vi "image_replacement.vi"(8 "buffer name":string, 10 "replacement":dbl[](array[numeric]), 11 "image in":T1(plugin-control)) -> (3 "image out":T1(plugin-control))   [LabVIEW 2017]
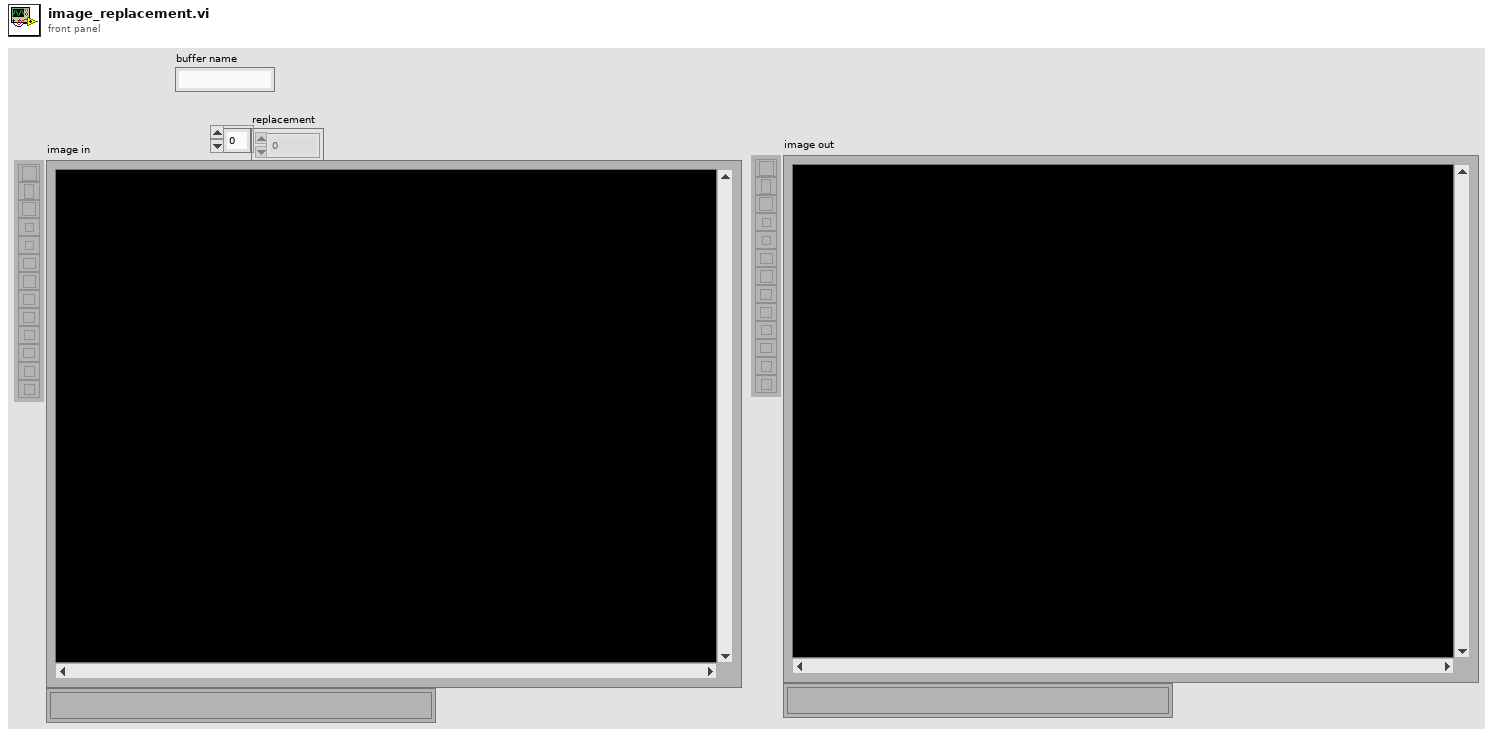
[diagram p1: front panel]
types:
  T1 = typedef "IMAQ Image.ctl" = refnum<image>
  T2 = typedef "Image Type" = u32
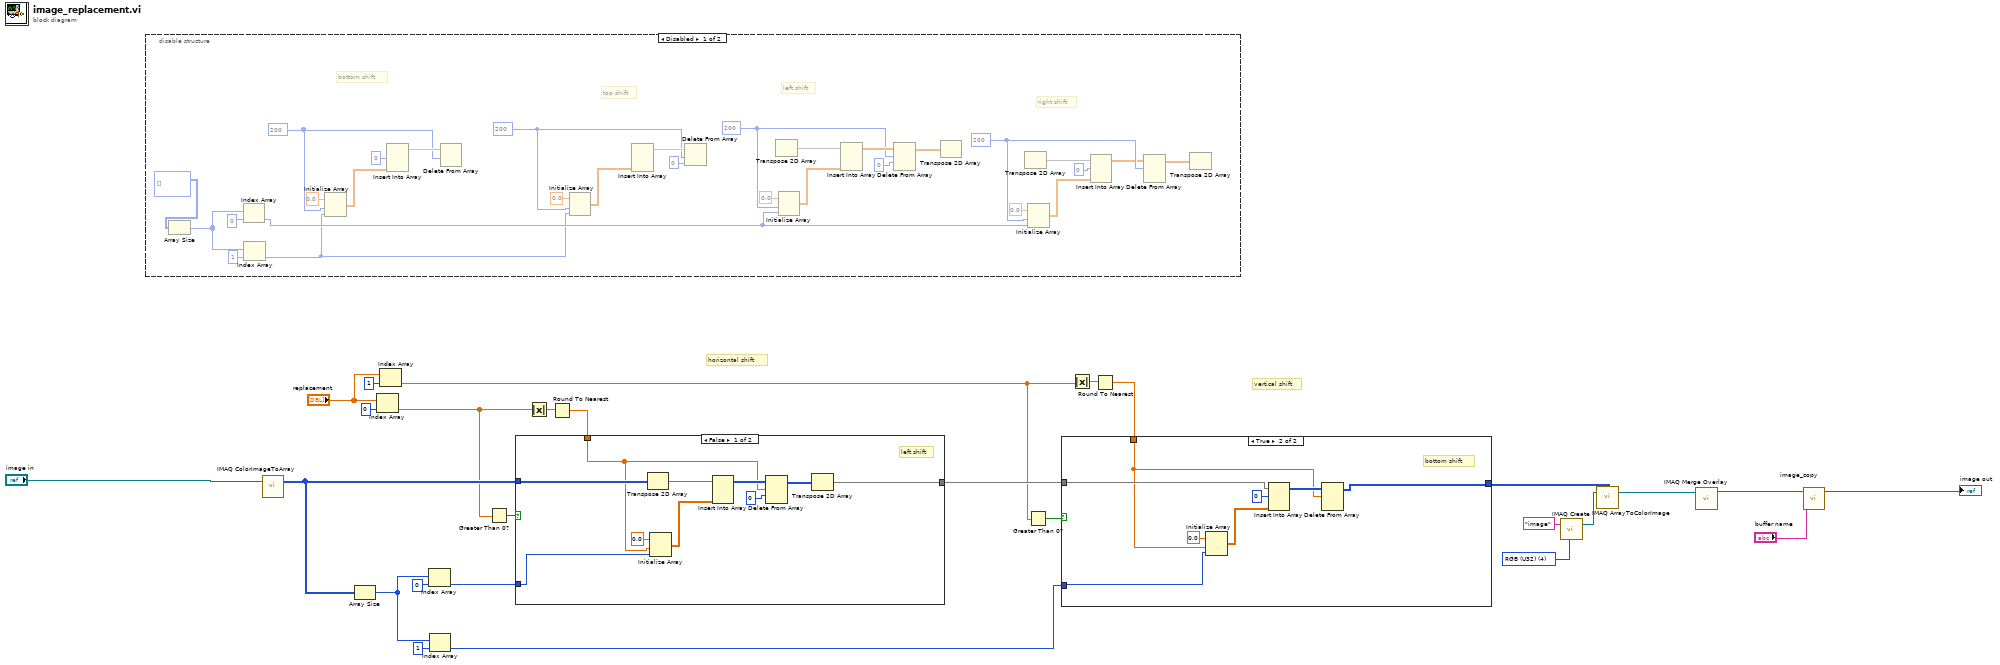
[diagram p0: block diagram]
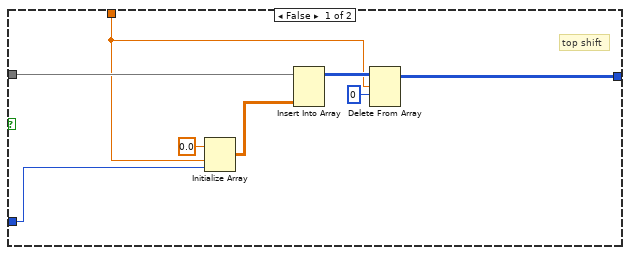
[diagram p2: hidden frame]
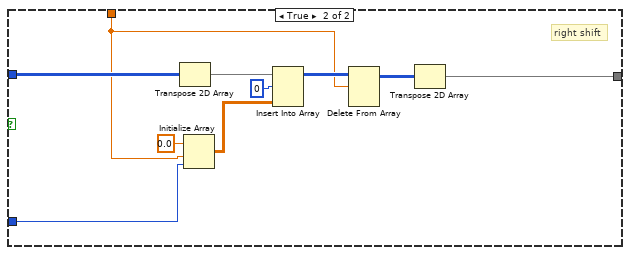
[diagram p3: hidden frame]
diagram:
  w26 = T2 4 items=["Grayscale (U8)", "Grayscale (I16)", "Grayscale (SGL)", "Complex (CSG)", "RGB (U32)", "HSL (U32)", "RGB (U64)", "Grayscale (U16)"] ("Image Type")
  # "vertical shift"
  # "horizontal shift"
  n1 = disable-structure shown="Disabled" {
    frame Disabled {
      w29 = 200
      w35 = 200
      w41 = 200
      w54 = 200
      # "right shift"
      # "left shift"
      # "top shift"
      # "bottom shift"
      n2 = Array Size(array=u32[][] [] ("Image Pixels (U32)")) -> (size(s)=w57:i32[])
      n3 = Index Array(array=w57, index=0) -> (element=w30:i32)
      n4 = Index Array(array=w57, index=1) -> (element=w28:i32)
      n5 = Initialize Array(0.0 ("element"), w29, w28) -> (w32:dbl[][])
      n6 = Insert Into Array(index (row)=0, new element=w32) -> (w33:dbl[])  [unwired: 2 in]
      n7 = Delete From Array(array=w33, length=w29) -> ()  [unwired: 1 in, 2 out]
      n8 = Initialize Array(0.0 ("element"), w35, w28) -> (w37:dbl[][])
      n9 = Insert Into Array(new element=w37) -> (w38:dbl[])  [unwired: 3 in]
      n10 = Delete From Array(array=w38, length=w35, index=0 ("index (row)")) -> ()  [unwired: 2 out]
      n11 = Transpose 2D Array() -> (transposed array=w44:dbl[][])  [unwired: 1 in]
      n12 = Initialize Array(0.0 ("element"), w41, w30) -> (w45:dbl[][])
      n13 = Insert Into Array(array=w44, new element=w45) -> (w43:dbl[][])  [unwired: 2 in]
      n14 = Delete From Array(array=w43, length=w41, index (row)=0) -> (array with subset deleted=w42:dbl[][])  [unwired: 1 in, 1 out]
      n15 = Transpose 2D Array(2D array=w42) -> ()  [unwired: 1 out]
      n16 = Transpose 2D Array() -> (transposed array=w51:dbl[][])  [unwired: 1 in]
      n17 = Initialize Array(0.0 ("element"), w54, w30) -> (w49:dbl[][])
      n18 = Insert Into Array(array=w51, index (row)=0, new element=w49) -> (w52:dbl[][])  [unwired: 1 in]
      n19 = Delete From Array(array=w52, length=w54) -> (array with subset deleted=w53:dbl[][])  [unwired: 2 in, 1 out]
      n20 = Transpose 2D Array(2D array=w53) -> ()  [unwired: 1 out]
    }
    frame Enabled {
    }
  }
  n21 = call "IMAQ ColorImageToArray"("Image"="image in") -> ("Image Pixels (U32)"=w18:u32[][])  [unwired: 3 in, 2 out]
  n22 = Array Size(array=w18) -> (size(s)=w21:i32[])
  n23 = Index Array(array="replacement", index=0) -> (element=w15:dbl)
  n24 = Index Array(array="replacement", index=1) -> (element=w7:dbl)
  n25 = Index Array(array=w21, index=0) -> (element=w17:i32)
  n26 = Index Array(array=w21, index=1) -> (element=w10:i32)
  n27 = Greater Than 0?(x=w15) -> (x > 0?=w16:bool)
  n28 = Absolute Value(x=w15) -> (abs(x)=w14:dbl)
  n29 = Round To Nearest(number=w14) -> (nearest integer value=w13:dbl)
  n30 = case shown="False" w16 {
    tunnel: w18 -> [w60 w71]
    tunnel: [w61 w70] -> w12
    tunnel: w17 -> [w59 w69]
    tunnel: w13 -> [w58 w68]
    frame False {
      # "left shift"
      n31 = Transpose 2D Array(2D array=w60) -> (transposed array=w64:u32[][])
      n32 = Initialize Array(0.0 ("element"), w58, w59) -> (w63:dbl[][])
      n33 = Insert Into Array(array=w64, new element=w63) -> (w65:u32[][])  [unwired: 2 in]
      n34 = Delete From Array(array=w65, length=w58, index (row)=0) -> (array with subset deleted=w66:u32[][])  [unwired: 1 in, 1 out]
      n35 = Transpose 2D Array(2D array=w66) -> (transposed array=w61:u32[][])
    }
    frame True {
      # "right shift"
      n36 = Transpose 2D Array(2D array=w71) -> (transposed array=w74:u32[][])
      n37 = Initialize Array(0.0 ("element"), w68, w69) -> (w76:dbl[][])
      n38 = Insert Into Array(array=w74, index (row)=0, new element=w76) -> (w73:u32[][])  [unwired: 1 in]
      n39 = Delete From Array(array=w73, length=w68) -> (array with subset deleted=w72:u32[][])  [unwired: 2 in, 1 out]
      n40 = Transpose 2D Array(2D array=w72) -> (transposed array=w70:u32[][])
    }
  }
  n41 = Greater Than 0?(x=w7) -> (x > 0?=w9:bool)
  n42 = Absolute Value(x=w7) -> (abs(x)=w8:dbl)
  n43 = Round To Nearest(number=w8) -> (nearest integer value=w6:dbl)
  n44 = case shown="True" w9 {
    tunnel: w12 -> [w81 w89]
    tunnel: [w80 w88] -> w11
    tunnel: w10 -> [w79 w87]
    tunnel: w6 -> [w78 w86]
    frame False {
      # "top shift"
      n45 = Initialize Array(0.0 ("element"), w78, w79) -> (w84:dbl[][])
      n46 = Insert Into Array(array=w81, new element=w84) -> (w83:u32[][])  [unwired: 2 in]
      n47 = Delete From Array(array=w83, length=w78, index (row)=0) -> (array with subset deleted=w80:u32[][])  [unwired: 1 in, 1 out]
    }
    frame True {
      # "bottom shift"
      n48 = Initialize Array(0.0 ("element"), w86, w87) -> (w92:dbl[][])
      n49 = Insert Into Array(array=w89, index (row)=0, new element=w92) -> (w91:u32[][])  [unwired: 1 in]
      n50 = Delete From Array(array=w91, length=w86) -> (array with subset deleted=w88:u32[][])  [unwired: 2 in, 1 out]
    }
  }
  n51 = call "IMAQ Create"("Image Name"="image", "Image Type"=w26) -> ("New Image"=w27:T1)  [unwired: 3 in, 1 out]
  n52 = call "IMAQ ArrayToColorImage"("Image Pixels (U32)"=w11, "Image"=w27) -> ("Image Out"=w5:T1)  [unwired: 3 in, 1 out]
  n53 = call "IMAQ Merge Overlay"("Image Src"=w5) -> ("Image Dst Out"=w2:T1)  [unwired: 9 in, 1 out]
  n54 = call "image_copy.vi"("buffer name"="buffer name", "image in"=w2) -> ("imgae out"=→"image out":T1)  [unwired: 9 in]
